vi "Make Hardware Resist and Temp Calls.vi"(8 "error in (no error)":errorcluster, 9 "CD Out Buf":dbl[](array[numeric]), 10 "CD In Buf":dbl[](array[numeric]), 11 "Engine Run Time Data in":T1) -> (0 "error out":errorcluster, 1 "CD Out Buf out":dbl[](array[numeric]), 3 "Engine Run Time Data out":T1)   [LabVIEW 2017, in "NI 272x Resistive Simulation Custom Device Engine.lvlib"]
uses:
  NI 272x Resistive Simulation Custom Device Engine.lvlib
  <instrlib>/ni272xReferenceVIs/ni272xReferenceVIs.llb/ni272x Write Temperature 1Chan 1Samp.vi
  <instrlib>/ni272xReferenceVIs/ni272xReferenceVIs.llb/ni272x Write Resistance 1Chan 1Samp.vi
  Controls/Channel Mode.ctl
  NI 272x Resistive Simulation Custom Device Shared.lvlib
  <instrlib>/ni272xReferenceVIs/ni272xReferenceVIs.llb/ni272x Callendar-Van Dusen RTD Parameters.ctl
  Controls/Compiled HW Channel.ctl
  Controls/Compiled Connect Channel.ctl
  Controls/Compiled Engine Data.ctl
  <instrlib>/ni272xReferenceVIs/ni272xReferenceVIs.llb/ni272x Reference.ctl
  Controls/Engine Run Time Data.ctl
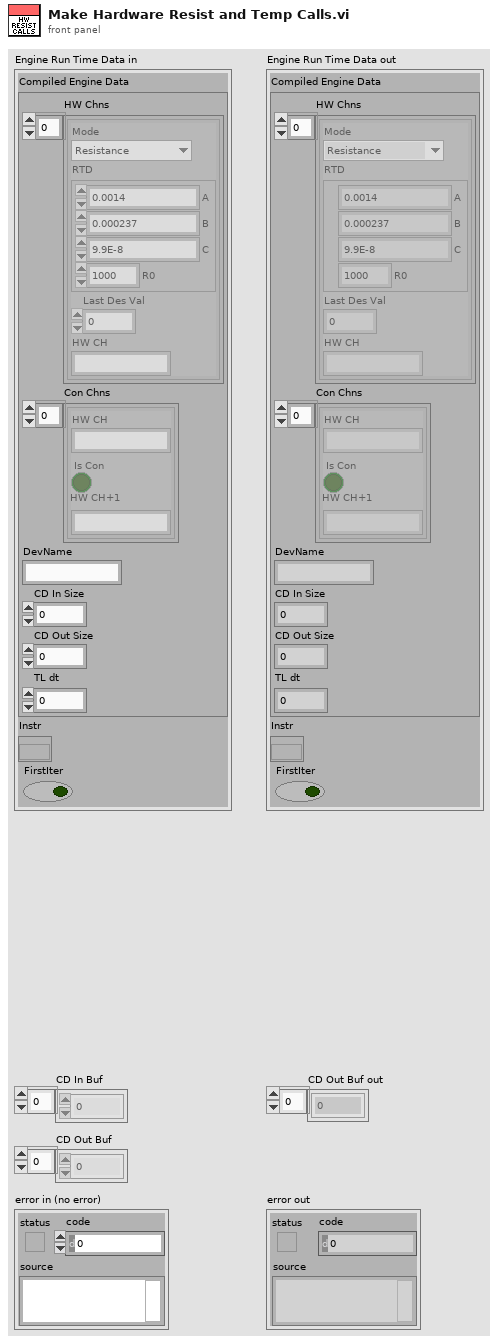
[diagram p1: front panel]
types:
  T1 = typedef "NI 272x Resistive Simulation Custom Device Engine.lvlib/Engine Run Time Data.ctl" = cluster{"Compiled Engine Data":T2, "Instr":T7, "FirstIter":bool}
  T2 = typedef "NI 272x Resistive Simulation Custom Device Shared.lvlib/Compiled Engine Data.ctl" = cluster{"HW Chns":T3[], "Con Chns":T6[], "DevName":string, "CD In Size":i32, "CD Out Size":i32, "TL dt":i64}
  T3 = typedef "NI 272x Resistive Simulation Custom Device Shared.lvlib/Compiled HW Channel.ctl" = cluster{"Mode":T4, "RTD":T5, "Last Des Val":dbl, "HW CH":string}
  T4 = typedef "NI 272x Resistive Simulation Custom Device Shared.lvlib/Channel Mode.ctl" = enum16{"Resistance", "RTD Temperature"}
  T5 = typedef "ni272x Callendar-Van Dusen RTD Parameters.ctl" = cluster{"A":dbl, "B":dbl, "C":dbl, "R0":dbl}
  T6 = typedef "NI 272x Resistive Simulation Custom Device Shared.lvlib/Compiled Connect Channel.ctl" = cluster{"HW CH":string, "Is Con":bool, "HW CH+1":string}
  T7 = typedef "ni272x Reference.ctl" = refnum<k20>
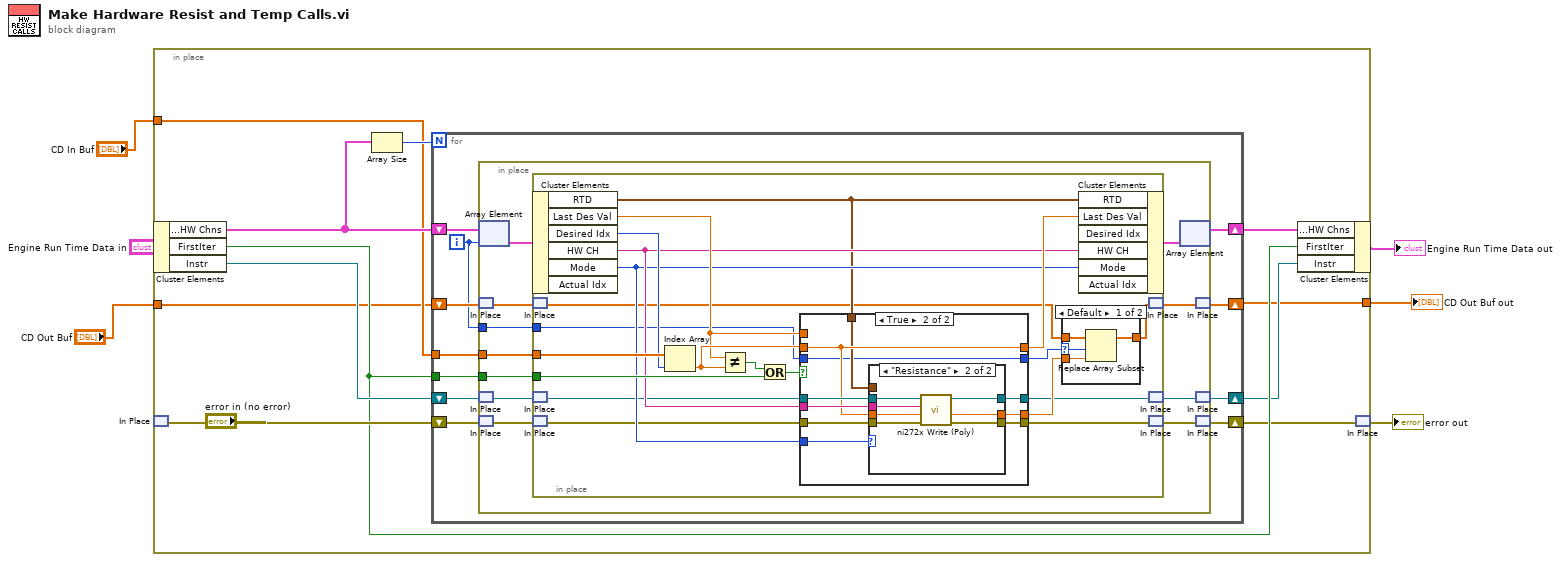
[diagram p0: block diagram]
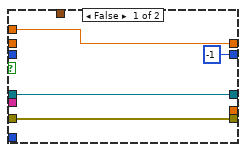
[diagram p3: hidden frame]
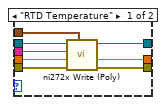
[diagram p4: hidden frame]
diagram:
  n1 = in-place {
    in-place-border: "CD In Buf" -> [w10]
    in-place-border: "CD Out Buf" -> [w9]
    in-place-border: [w8] -> w1
    n2 = in-place-cluster #1("Engine Run Time Data in") -> ("Compiled Engine Data.HW Chns"=w15:T3[], "FirstIter"=w13:bool, "Instr"=w18:T7)
    n3 = in-place-match #2("error in (no error)") -> (w17:errorcluster)
    n4 = Array Size(array=w15) -> (size(s)=w16:i32)
    n5 = for {
      N: w16 -> [_]
      tunnel: w10 -> [w28]
      tunnel: w13 -> [w27]
      shift-right: [w21] -> w12
      shift-left: w18 -> [w22]
      shift-right: [w23] -> w8
      shift-left: w9 -> [w24]
      shift-right: [w25] -> w11
      shift-left: w17 -> [w26]
      shift-right: [w20] -> w14
      shift-left: w15 -> [w29]
      i -> [w19]
      n6 = in-place {
        in-place-border: w28 -> [w39]
        in-place-border: w27 -> [w38]
        in-place-border: w19 -> [w30]
        n7 = in-place-array #3(w29, w19) -> (w40:T3)
        n8 = in-place-match #4(w24) -> (w34:dbl[])
        n9 = in-place-match #5(w22) -> (w32:T7)
        n10 = in-place-match #6(w26) -> (w37:errorcluster)
        n11 = in-place {
          in-place-border: w39 -> [w60]
          in-place-border: w38 -> [w58]
          in-place-border: w30 -> [w41]
          n12 = in-place-cluster #7(w40) -> ("RTD"=w50:T5, "Last Des Val"=w55:dbl, "Desired Idx"=w54:i32, "HW CH"=w52:string, "Mode"=w51:T4)  [unwired: 1 out]
          n13 = in-place-match #8(w34) -> (w45:dbl[])
          n14 = in-place-match #9(w32) -> (w43:T7)
          n15 = in-place-match #10(w37) -> (w48:errorcluster)
          n16 = Index Array(array=w60, index=w54) -> (element=w56:dbl)
          n17 = Not Equal?(x=w55, y=w56) -> (x != y?=w59:bool)
          n18 = Or(x=w59, y=w58) -> (x .or. y?=w57:bool)
          n19 = case shown="True" w57 {
            tunnel: w56 -> [_ w75]
            tunnel: w55 -> [w69 _]
            tunnel: [w69 w75] -> w53
            tunnel: w51 -> [_ w79]
            tunnel: w52 -> [_ w76]
            tunnel: w48 -> [w67 w78]
            tunnel: w43 -> [w66 w77]
            tunnel: w50 -> [_ w74]
            tunnel: [_ w73] -> w49
            tunnel: [w67 w72] -> w47
            tunnel: [w66 w71] -> w42
            tunnel: w41 -> [_ w70]
            tunnel: [-1 ("Actual Idx") w70] -> w46
            frame False {
            }
            frame True {
              n20 = case shown="\"Resistance\"" w79 {
                tunnel: w78 -> [w87 w94]
                tunnel: w77 -> [w86 w93]
                tunnel: w76 -> [w85 w92]
                tunnel: w75 -> [w84 w91]
                tunnel: w74 -> [w83 _]
                tunnel: [w82 w90] -> w72
                tunnel: [w81 w89] -> w71
                tunnel: [w80 w88] -> w73
                frame "RTD Temperature" {
                  n21 = call-poly <instrlib>:"ni272x Write (Poly).vi"("Callendar-Van Dusen RTD parameters"=w83, "error in (no error)"=w87, "requested temperature (degrees Celsius)"=w84, "resistor channel"=w85, "instrument handle"=w86) -> ("error out"=w82:errorcluster, "coerced temperature (degrees Celsius)"=w80:dbl, "instrument handle out"=w81:T7)  [unwired: 4 out]
                }
                frame "Resistance" {
                  n22 = call-poly <instrlib>:"ni272x Write (Poly).vi"("error in (no error)"=w94, "requested resistance (ohms)"=w91, "resistor channel"=w92, "instrument handle"=w93) -> ("error out"=w90:errorcluster, "coerced resistance (ohms)"=w88:dbl, "instrument handle out"=w89:T7)  [unwired: 1 in, 4 out]
                }
              }
            }
          }
          n23 = case shown="Default" w46 {
            selector: w46 -> [w63 _]
            tunnel: w45 -> [w64 w65]
            tunnel: w49 -> [w62 _]
            tunnel: [w61 w65] -> w44
            frame Default {
              n24 = Replace Array Subset(array=w64, new element=w62, index=w63) -> (w61:dbl[])
            }
            frame -1 {
            }
          }
          n25 = in-place-cluster #7("RTD"=w50, "Last Des Val"=w53, "HW CH"=w52, "Mode"=w51) -> (w35:T3)  [unwired: 2 in]
          n26 = in-place-match #8(w44) -> (w33:dbl[])
          n27 = in-place-match #9(w42) -> (w31:T7)
          n28 = in-place-match #10(w47) -> (w36:errorcluster)
        }
        n29 = in-place-array #3(w35) -> (w20:T3[])  [unwired: 1 out]
        n30 = in-place-match #4(w33) -> (w23:dbl[])
        n31 = in-place-match #5(w31) -> (w21:T7)
        n32 = in-place-match #6(w36) -> (w25:errorcluster)
      }
    }
    n33 = in-place-cluster #1("Compiled Engine Data.HW Chns"=w14, "FirstIter"=w13, "Instr"=w12) -> (→"Engine Run Time Data out":T1)
    n34 = in-place-match #2(w11) -> (→"error out":errorcluster)
  }
  "CD Out Buf out" <- w1
